vi "GeneratorSemnalProject.vi"() -> ()   [LabVIEW 2024]
uses:
  <vilib>/DAQmx/write.llb/DAQmx Write (Analog 1D Wfm NChan NSamp).vi
  <vilib>/DAQmx/create/channels.llb/DAQmx Create Channel (AO-Voltage-Basic).vi
  <vilib>/DAQmx/configure/timing.llb/DAQmx Timing (Sample Clock).vi
  <vilib>/DAQmx/miscellaneous.llb/DAQmx Fill In Error Info.vi
  <resource>/objmgr/daqmx.rc
  <vilib>/measure/NI_MABase.lvlib
panel:
  in  "Duty Cycle CH1":dbl=50.0 format="%0.2f"
  in  "Duty Cycle CH2":dbl=50.0 format="%0.2f"
  in  "TURN OFF":bool
  in  "CH2 I/O":bool
  in  "CH1 I/O":bool
  out "error out":errorcluster
  out "CH2 Output":waveform(dbl)(graph)
  out "CH1 Output":waveform(dbl)(graph)
  in  "Offset CH2":dbl format="%0.2p"
  in  "Tipul Semnalului CH2":T1(ring)
  in  "Amplitudine CH2":i32
  in  "Frecventa CH2":dbl
  in  "Offset CH1":dbl format="%0.2p"
  in  "Tipul Semnalului CH1":T1(ring)
  in  "Amplitudine CH1":i32
  in  "Frecventa CH1":dbl
  in  "Frecventa De Esantionare":dbl=1000.0 format="%0.2f"
  in  "Numar Esantionari":i32
  in  "Valoare Max (valoare fizica)":dbl(slide)=10.0 scale=0.01..10.0
  in  "Valoare Min (valoare fizica)":dbl(slide)=-10.0 scale=0.0..-10.0
  in  "Canal/Canale Out Analogic":tag
  in  "error in":errorcluster
  # "Generator de semnal\n                                        Proiect SAM - Isachi Mihai - 6503\n                                                                 2024"
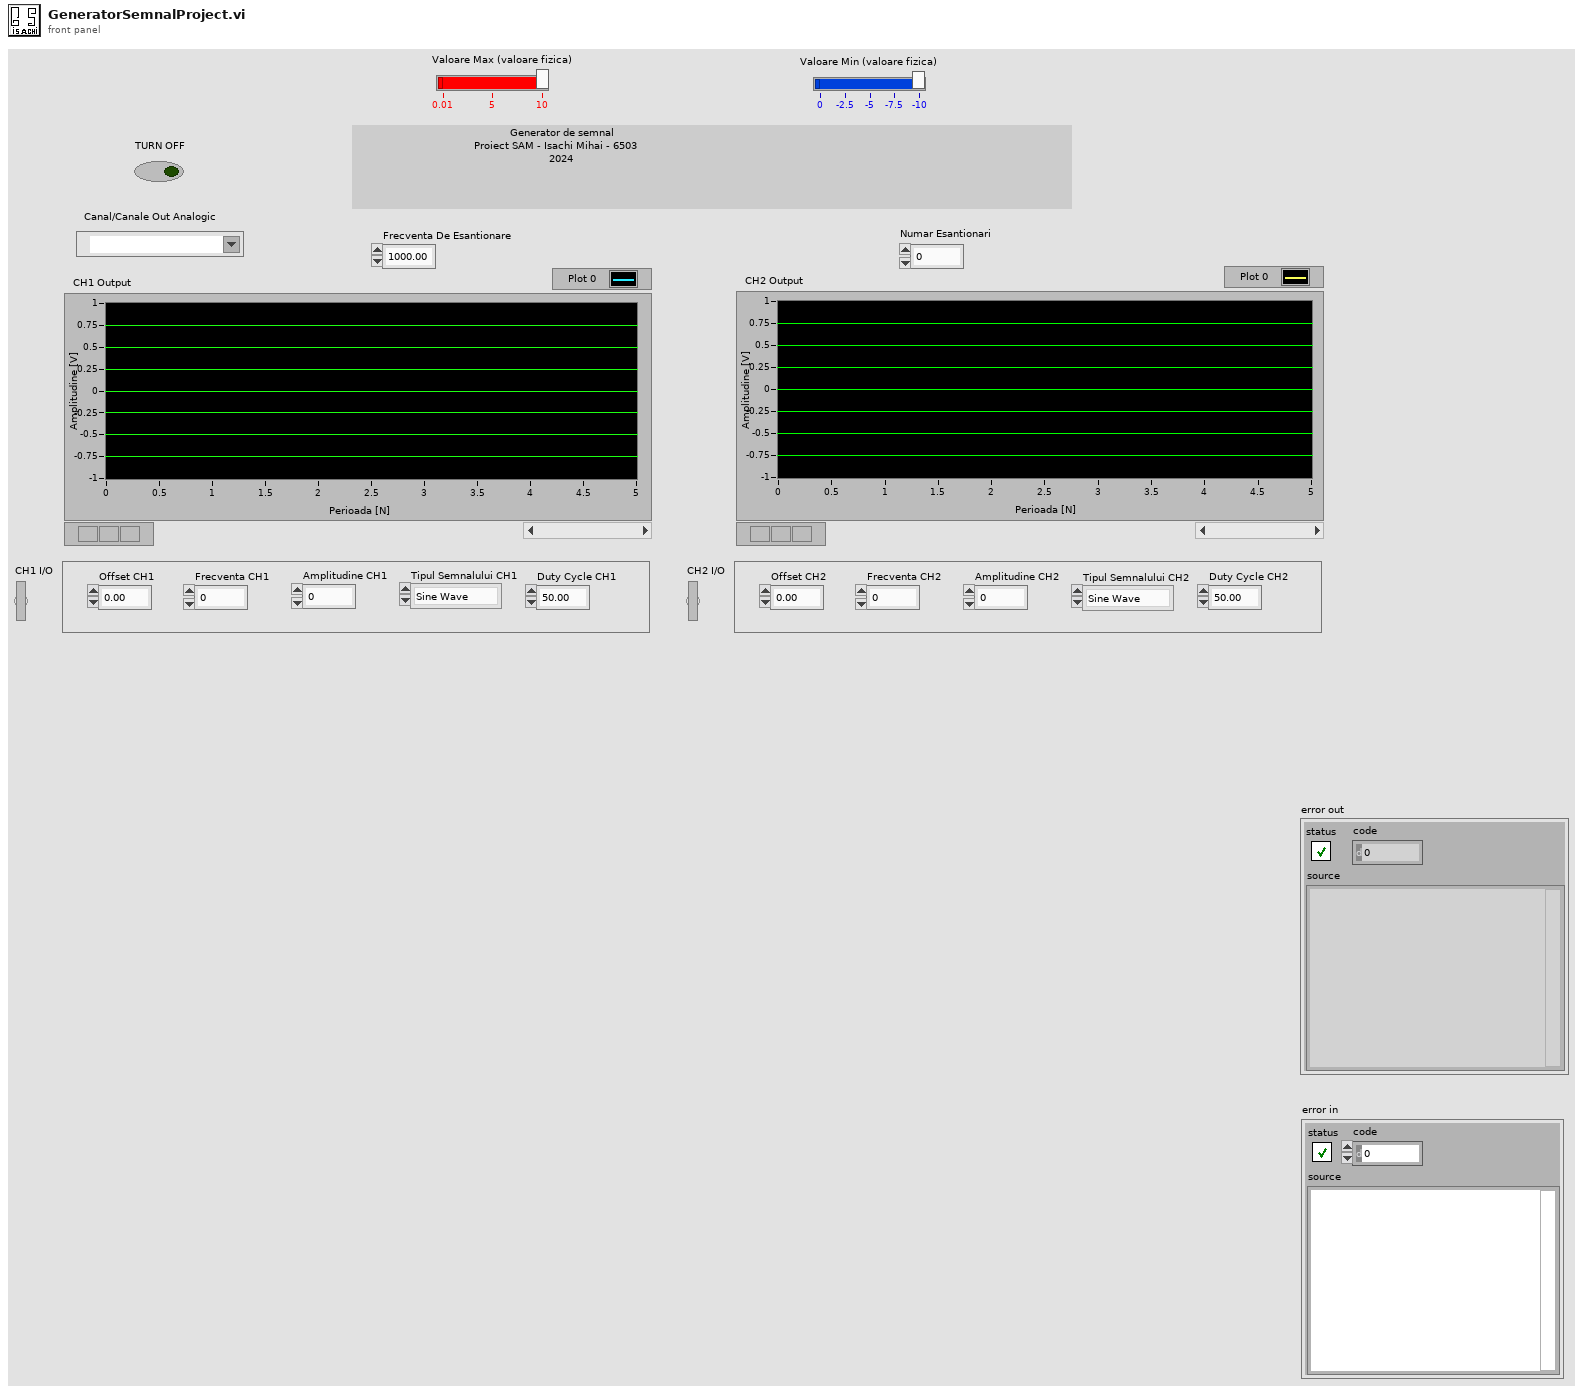
[diagram p1: front panel]
types:
  T1 = enum16{"Sine Wave", "Triangle Wave", "Square Wave", "Sawtooth Wave"}
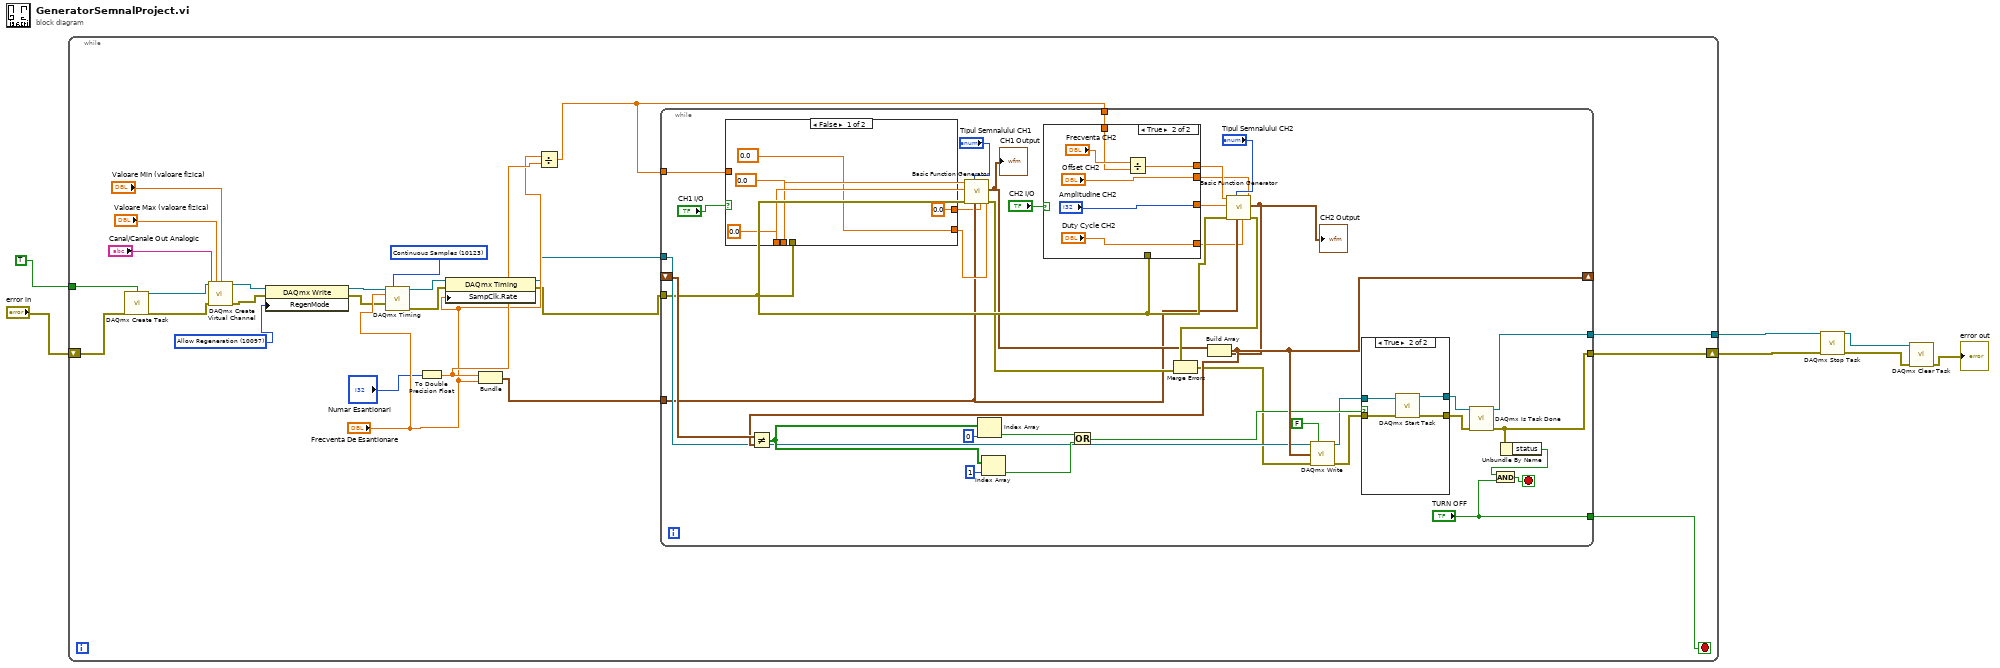
[diagram p0: block diagram]
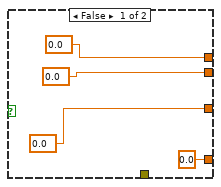
[diagram p3: hidden frame]
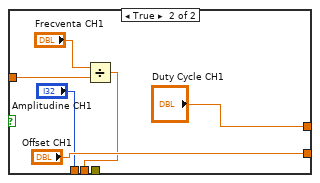
[diagram p4: hidden frame]
diagram:
  n1 = while {
    tunnel: [w32] -> w4
    tunnel: TRUE ("auto cleanup") -> [w10]
    shift-right: [w31] -> w3
    shift-left: "error in" -> [w9]
    stop <- w8 stop-if-true
    w16 = 10097 items=["Allow Regeneration"=10097, "Do Not Allow Regeneration"=10158] ("RegenMode")
    w15 = 10123 items=["Finite Samples"=10178, "Continuous Samples"=10123, "Hardware Timed Single Point"=12522] ("sample mode")
    n2 = call <vilib>:"DAQmx Create Task.vi"("auto cleanup"=w10, "error in"=w9) -> ("task out"=w21:refnum<k21>, "error out"=w22:errorcluster)  [unwired: 12 in]
    n3 = call-poly <vilib>:"DAQmx Create Virtual Channel.vi"("task in"=w21, "maximum value"="Valoare Max (valoare fizica)", "minimum value"="Valoare Min (valoare fizica)", "physical channels"="Canal/Canale Out Analogic", "error in"=w22) -> ("task out"=w23:refnum<k21>, "error out"=w25:errorcluster)  [unwired: 9 in]
    n4 = property class="DAQmx Write"(reference=w23, error in=w25, "RegenMode"=w16) -> (reference out=w24:refnum<k21>, error out=w26:errorcluster)
    n5 = call-poly <vilib>:"DAQmx Timing.vi"("task/channels in"=w24, "sample mode"=w15, "rate"="Frecventa De Esantionare", "error in"=w26) -> ("task out"=w27:refnum<k21>, "error out"=w28:errorcluster)  [unwired: 10 in]
    n6 = To Double Precision Float(number="Numar Esantionari") -> (double precision float=w30:dbl)
    n7 = property class="DAQmx Timing"(reference=w27, error in=w28, "SampClk.Rate"="Frecventa De Esantionare") -> (reference out=w13:refnum<k21>, error out=w12:errorcluster)
    n8 = Bundle(w30, "Frecventa De Esantionare"="Frecventa De Esantionare") -> (w11:cluster{dbl, "Frecventa De Esantionare":dbl})  [unwired: 1 in]
    n9 = Divide(x="Frecventa De Esantionare", y=w30) -> (x/y=w14:dbl)
    n10 = while {
      tunnel: w11 -> [w47]
      tunnel: w13 -> [w62]
      shift-right: [w69] -> _
      shift-left: _ -> [w70]
      tunnel: [w37] -> w32
      tunnel: [w36] -> w31
      tunnel: w12 -> [w58]
      tunnel: w14 -> [w46]
      tunnel: w14 -> [w45]
      tunnel: ["TURN OFF"] -> w8
      stop <- w38 stop-if-true
      n11 = case shown="False" "CH1 I/O" {
        tunnel: w58 -> [_ _]
        tunnel: [0.0 ("frequency") "Offset CH1"] -> w53
        tunnel: [0.0 ("offset") "Amplitudine CH1"] -> w52
        tunnel: [0.0 ("amplitude") w94] -> w51
        tunnel: w46 -> [_ w96]
        tunnel: [0.0 ("Duty Cycle CH1") "Duty Cycle CH1"] -> w34
        frame False {
        }
        frame True {
          n12 = Divide(x="Frecventa CH1", y=w96) -> (x/y=w94:dbl)
        }
      }
      n13 = call <vilib>:"Basic Function Generator.vi"("offset"=w53, "square wave duty cycle (%)"=w34, "sampling info"=w47, "signal type"="Tipul Semnalului CH1", "error in (no error)"=w58, "amplitude"=w52, "frequency"=w51) -> ("error out"=w50:errorcluster, "signal out"=w49:waveform(dbl))  [unwired: 2 in, 1 out]
      "CH1 Output" <- w49
      n14 = case shown="True" "CH2 I/O" {
        tunnel: w58 -> [_ _]
        tunnel: w45 -> [_ w87]
        tunnel: [0.0 ("frequency") w86] -> w44
        tunnel: [0.0 ("offset") "Amplitudine CH2"] -> w43
        tunnel: [0.0 ("amplitude") "Offset CH2"] -> w42
        tunnel: [0.0 ("square wave duty cycle (%)") "Duty Cycle CH2"] -> w35
        frame False {
        }
        frame True {
          n15 = Divide(x="Frecventa CH2", y=w87) -> (x/y=w86:dbl)
        }
      }
      n16 = call <vilib>:"Basic Function Generator.vi"("offset"=w42, "square wave duty cycle (%)"=w35, "sampling info"=w47, "signal type"="Tipul Semnalului CH2", "error in (no error)"=w58, "amplitude"=w43, "frequency"=w44) -> ("error out"=w56:errorcluster, "signal out"=w55:waveform(dbl))  [unwired: 2 in, 1 out]
      "CH2 Output" <- w55
      n17 = Merge Errors(w56, w50) -> (w61:errorcluster)
      n18 = Build Array(w49, w55) -> (w69:waveform(dbl)[])
      n19 = Not Equal?(x=w70, y=w69) -> (x != y?=w66:bool[])
      n20 = Index Array(array=w66, index=0) -> (element=w65:bool)
      n21 = Index Array(array=w66, index=1) -> (element=w64:bool)
      n22 = Or(x=w65, y=w64) -> (x .or. y?=w63:bool)
      n23 = call-poly <vilib>:"DAQmx Write.vi"("task/channels in"=w62, "auto start"=FALSE, "data"=w69, "error in"=w61) -> ("task out"=w60:refnum<k21>, "error out"=w59:errorcluster)  [unwired: 9 in, 1 out]
      n24 = case shown="True" w63 {
        tunnel: w59 -> [w73 w77]
        tunnel: w60 -> [w74 w78]
        tunnel: [w74 w76] -> w41
        tunnel: [w73 w75] -> w40
        frame False {
        }
        frame True {
          n25 = call <vilib>:"DAQmx Start Task.vi"("task/channels in"=w78, "error in"=w77) -> ("task out"=w76:refnum<k21>, "error out"=w75:errorcluster)  [unwired: 12 in]
        }
      }
      n26 = call <vilib>:"DAQmx Is Task Done.vi"("task/channels in"=w41, "error in"=w40) -> ("task out"=w37:refnum<k21>, "error out"=w36:errorcluster)  [unwired: 11 in, 1 out]
      n27 = Unbundle By Name(w36) -> ("status"=w39:bool)
      n28 = And(x=w39, y="TURN OFF") -> (x .and. y?=w38:bool)
    }
  }
  n29 = call <vilib>:"DAQmx Stop Task.vi"("task/channels in"=w4, "error in"=w3) -> ("task out"=w6:refnum<k21>, "error out"=w5:errorcluster)  [unwired: 12 in]
  n30 = call <vilib>:"DAQmx Clear Task.vi"("task in"=w6, "error in"=w5) -> ("error out"=→"error out":errorcluster)  [unwired: 13 in]
